vi "3.0.0_Power_Tunings & AW_Performance_Test_ECO_&_BOOST.vi"(7 "Data in":T1, 8 "error in (no error)":errorcluster, 9 "AllControls In":T2, 10 "?":T4, 11 "Message Queue out":T5) -> (0 "error out":errorcluster, 1 "Flow":string, 2 "Data":T4, 3 "Message Queue Out":T5, 5 "Data out":T1)   [LabVIEW 2017]
uses:
  Depends/AMC/subVIs/TypeDefs/amc_Message Queue.ctl
  Depends/AMC/subVIs/TypeDefs/amc_Message.ctl
  Depends/Tools/Keyed Array/Tools_KeyedArray KeyedArray.ctl
  Ctrls/Data.ctl
  DIPC 692 Daemon API/typdef/airwatt tune parameter.ctl
  Ctrls/AllControls.ctl
  Ctrls/CSV_Data.ctl
  DIPC 692 Daemon API/typdef/calibration.ctl
panel:
  out "Array":T3[](array[typedef])
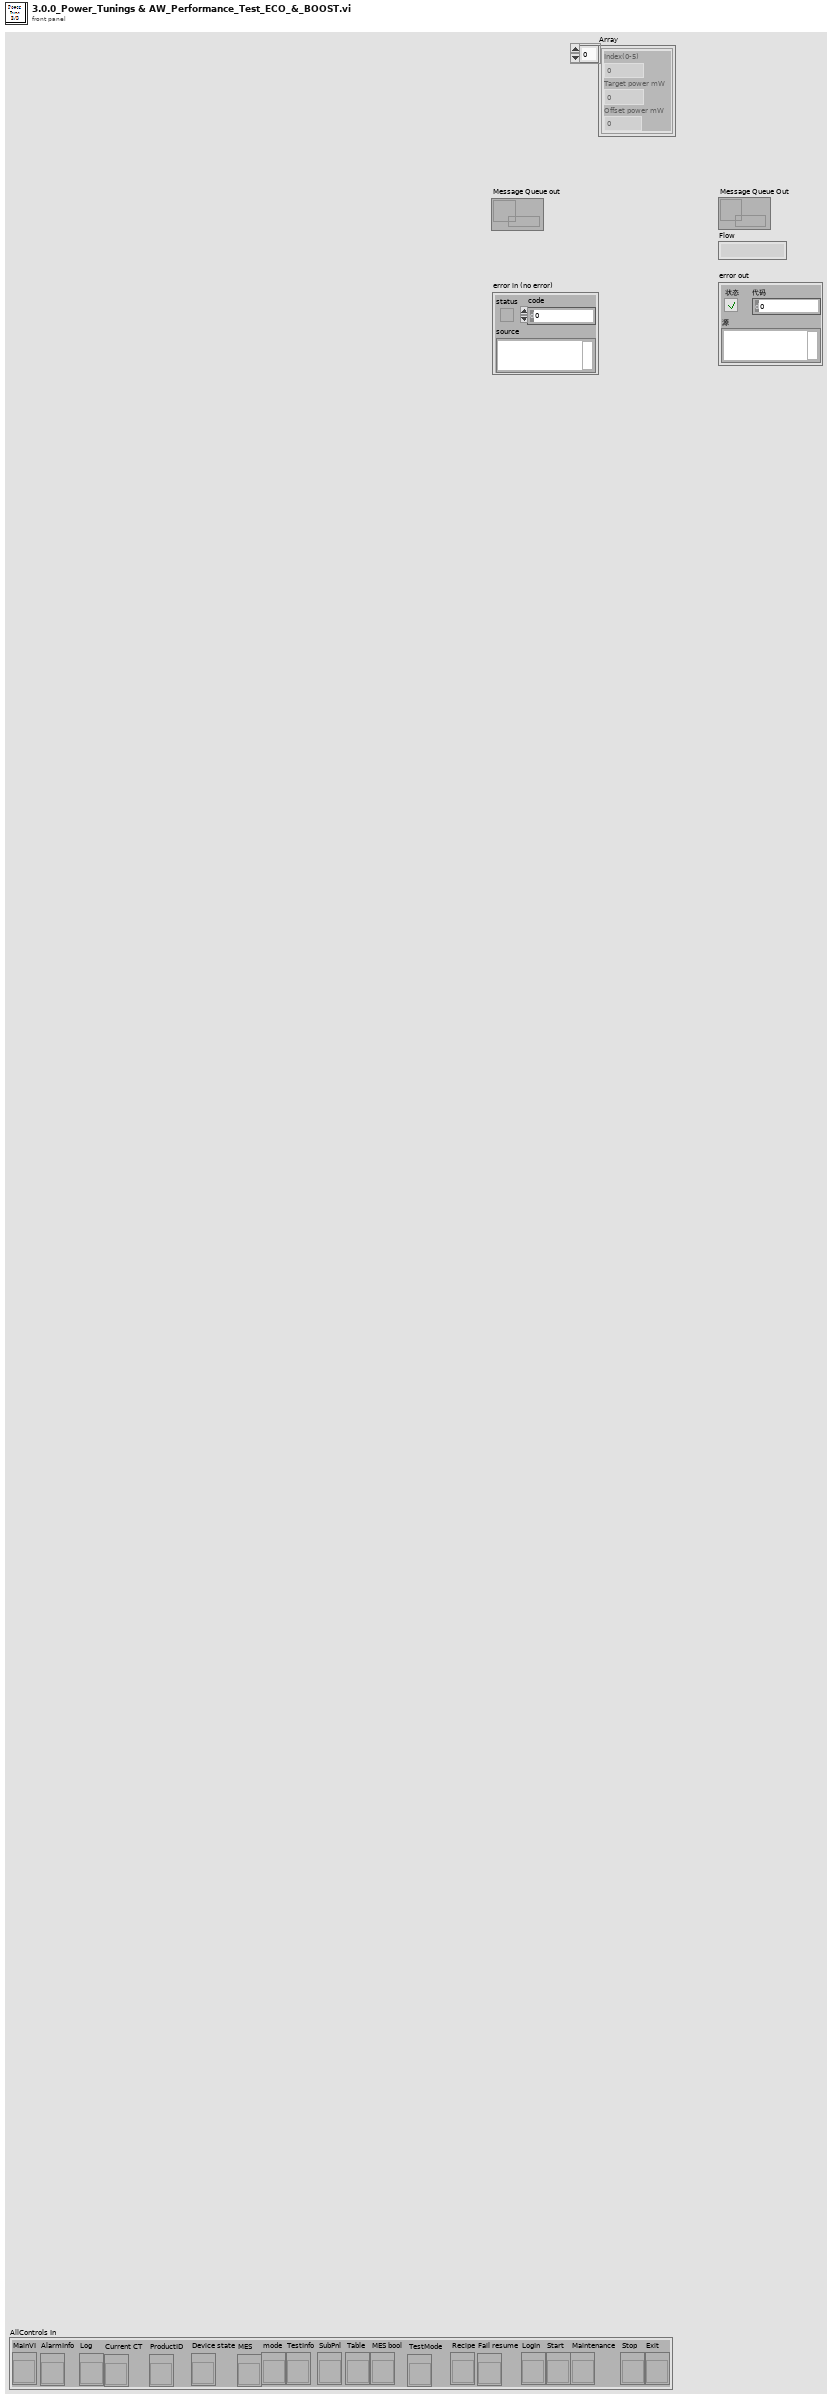
[diagram p1: front panel]
types:
  T1 = typedef "CSV_Data.ctl" = cluster{"Initialisation":cluster{"LMT - Connect UUT (con COM)":string, "LMT - Software Version (rrel)":string, "LMT - Write SKU file (wskuc)":string, "LMT - SKU file name":string, "Connect UUT DDM":string, "Read DDM EOL Timestamp - Mode":string, "Read DDM EOL Timestamp - Timestamp":string, "Read DDM EOL Timestamp - Rig ID":string, "Read DDM EOL Timestamp - Passmark ID":string, "Read DDM EOL Timestamp - Passmark Rev":string, "Software Version before flashing":string, "Read Hardware Serial":string, "UUT DDM SN":string, "Compare DDM SN with MES SN":string, "Backup PCBA Calibration EEPROM Response - CAL":string, "Flash Firmware Version":string, "Check SW Version":string, "Read DDM SW Version after flashing":string, "Set SKU Config":string, "Ready Status":string, "Set Device Mode to EOL":string, "DDM Parameter - Voltage":string, "DDM Parameter - Current":string, "DDM Parameter - Power":string, "DDM Parameter - Speed":string, "DDM Parameter - Pressure":string, "Tester Parameter - Voltage":string, "Tester Parameter - Current":string, "Tester Parameter - Power":string, "Tester Parameter - Ambient Pressure":string, "Tester Parameter - Ambient Temperature":string, "Calculated Parameter - DDM Pressure Corrected":string, "Calculated Parameter - DDM Real Power":string, "Calculated Parameter - Delta V":string}, "BEMF_Calibration":cluster{"Calibration Result - eol_cold_bemf_temp":string, "DDM Ambient Temp":string, "Restriction Plate Diameter":string, "Calibration Result - eol_bemf_mp_cold_coef_a":string, "Calibration Result - eol_bemf_mp_cold_coef_b":string, "Calibration Result - eol_bemf_mp_cold_coef_c":string, "Calibration Result - eol_bemf_lsi_cold_ref_coeffs":string, "Get - Calibration Result - eol_bemf_lsi_speed":string, "Get - Calibration Result - eol_bemf_lsi_integral_0":string, "Calibration Result - eol_bemf_lsi_integral_1":string, "Get - Calibration Result - eol_bemf_lsi_integral_2":string, "Get - Calibration Result - eol_cold_bemf":string, "Get - Calibration Result - eol_cold_bemf_fisf":string, "Finalise Calibration":string, "Compare -Calibration Result - eol_cold_bemf":string, "Compare -Calibration Result - eol_cold_bemf_fisf":string}, "ECO":cluster{"Reset Power Tune":string, "Reset BEMF FISF Calibration":string, "Restriction Plate Diameter":string, "ECO - Stabilisation Time":string, "ECO - DDM Parameter - Voltage":string, "ECO - DDM Parameter - Current":string, "ECO - DDM Parameter - Power":string, "ECO - DDM Parameter - Measured Power":string, "ECO - DDM Parameter - Speed":string, "ECO - DDM Parameter - Pressure":string, "ECO - Tester Parameter - Voltage":string, "ECO - Tester Parameter - Current":string, "ECO - Tester Parameter - Power":string, "ECO - Tester Parameter - Ambient Pressure":string, "ECO - Tester Parameter - Ambient Temperature":string, "ECO - Tester Parameter - Ambient Humidity":string, "ECO - Calculated Parameter - DDM Pressure Corrected":string, "ECO - Calculated Parameter - DDM Real Power":string, "ECO - Calculated Parameter - Delta V":string, "ECO - Calculated Parameter - Flowrate":string, "ECO - Calculated Parameter - Airwatt":string, "ECO - Formula":string, "PT ECO - Power Tune Mode Status":string}, "BOOST":cluster{"Restriction Plate Diameter":string, "BOOST - Stabilisation Time":string, "BOOST - DDM Parameter - Voltage":string, "BOOST - DDM Parameter - Current":string, "BOOST - DDM Parameter - Power":string, "BOOST - DDM Parameter - Measured Power":string, "BOOST - DDM Parameter - Speed":string, "BOOST - DDM Parameter - Pressure":string, "BOOST - Tester Parameter - Voltage":string, "BOOST - Tester Parameter - Current":string, "BOOST - Tester Parameter - Power":string, "BOOST - Tester Parameter - Ambient Pressure":string, "BOOST - Tester Parameter - Ambient Temperature":string, "BOOST - Tester Parameter - Ambient Humidity":string, "BOOST - Calculated Parameter - DDM Pressure Corrected":string, "BOOST - Calculated Parameter - DDM Real Power":string, "BOOST - Calculated Parameter - Delta V":string, "BOOST - Calculated Parameter - Flowrate":string, "BOOST - Calculated Parameter - Airwatt":string, "BOOST - Get AM Presence":string, "Air Muscle Turn Off Status":string, "BOOST - Air Muscle Calculated Parameter - Airwatt B":string, "BOOST - Air Muscle Calculate Airwatt Delta":string, "PT BOOST - Power Tune Mode Status":string, "Finalise Calibration":string, "ECO - Get AW Calibration value":string, "BOOST - Get AW Calibration value":string}, "MAX":cluster{"Restriction Plate Diameter":string, "MAX - Stabilisation Time":string, "Get Average Delta Tmag (LSIdelta_FISFdelta_LSItmag_FISFtmag_IIRtmag)":string, "Get Average Delta Tmag FISF":string, "MAX - DDM Parameter - Voltage":string, "MAX - DDM Parameter - Current":string, "MAX - DDM Parameter - Power":string, "MAX - DDM Parameter - Measured Power":string, "MAX - DDM Parameter - Speed":string, "MAX - DDM Parameter - Pressure":string, "MAX - Tester Parameter - Voltage":string, "MAX - Tester Parameter - Current":string, "MAX - Tester Parameter - Power":string, "MAX - Tester Parameter - Ambient Pressure":string, "MAX - Tester Parameter - Ambient Temperature":string, "MAX - Tester Parameter - Ambient Humidity":string, "MAX - Calculated Parameter - DDM Pressure Corrected":string, "MAX - Calculated Parameter - DDM Real Power":string, "MAX - Calculated Parameter - Delta V":string, "MAX - Calculated Parameter - Flowrate":string, "MAX - Calculated Parameter - Airwatt":string, "MAX_FISF_Check_Average_Delta_Tmag":string, "MAX - FISF - BEMF Finetune Result":string, "MAX tune - Delta P1":string, "MAX tune - Calculated Parameter - Airwatt":string, "Calculate Delta Airwatts - MAX finetune - Delta P2":string, "MAX finetune - DDM Parameter - Voltage":string, "MAX finetune - DDM Parameter - Current":string, "MAX finetune - DDM Parameter - Power":string, "MAX finetune - DDM Parameter - Measured Power":string, "MAX finetune - DDM Parameter - Speed":string, "MAX finetune - DDM Parameter - Pressure":string, "MAX finetune - Tester Parameter - Voltage":string, "MAX finetune - Tester Parameter - Current":string, "MAX finetune - Tester Parameter - Power":string, "MAX finetune - Tester Parameter - Ambient Pressure":string, "MAX finetune - Tester Parameter - Ambient Temperature":string, "MAX finetune - Tester Parameter - Ambient Humidity":string, "MAX finetune - Calculated Parameter - DDM Pressure Corrected":string, "MAX finetune - Calculated Parameter - DDM Real Power":string, "MAX finetune - Calculated Parameter - Delta V":string, "MAX finetune - Calculated Parameter - Flowrate":string, "MAX finetune - Calculated Parameter - Airwatt":string, "Check Derate Result":string, "Delta Tmag FISF":string, "Get Hot BEMF Result":string, "Calculate delta Pressure":string, "Finalise Calibration":string, "Calculate & Check Delta BEMF":string, "Delta P Airwatts Value":string}, "LL":cluster{"DDM Ambient Temp":string, "Restriction Plate Diameter":string, "LL - DDM Parameter - Voltage":string, "LL - DDM Parameter - Current":string, "LL - DDM Parameter - Power":string, "LL - DDM Parameter - Measured Power":string, "LL - DDM Parameter - Speed":string, "LL - DDM Parameter - Pressure":string, "LL - Tester Parameter - Voltage":string, "LL - Tester Parameter - Current":string, "LL - Tester Parameter - Power":string, "LL - DDM Real Power":string, "LL - Calibrate Task Detect LL":string}, "HL":cluster{"HL - DDM Parameter - Voltage":string, "HL - DDM Parameter - Current":string, "HL - DDM Parameter - Power":string, "HL - DDM Parameter - Measured Power":string, "HL - DDM Parameter - Speed":string, "HL - DDM Parameter - Pressure":string, "HL - Tester Parameter - Voltage":string, "HL - Tester Parameter - Current":string, "HL - Tester Parameter - Power":string, "HL - DDM Real Power":string, "HL - Calibrate Task Detect HL":string}, "LH":cluster{"Restriction Plate Diameter":string, "LH - DDM Parameter - Voltage":string, "LH - DDM Parameter - Current":string, "LH - DDM Parameter - Power":string, "LH - DDM Parameter - Measured Power":string, "LH - DDM Parameter - Speed":string, "LH - DDM Parameter - Pressure":string, "LH - Tester Parameter - Voltage":string, "LH - Tester Parameter - Current":string, "LH - Tester Parameter - Power":string, "LH - DDM Real Power":string, "LH - Calibrate Task Detect LH":string}, "HH":cluster{"HH - DDM Parameter - Voltage":string, "HH - DDM Parameter - Current":string, "HH - DDM Parameter - Power":string, "HH - DDM Parameter - Measured Power":string, "HH - DDM Parameter - Speed":string, "HH - DDM Parameter - Pressure":string, "HH - Tester Parameter - Voltage":string, "HH - Tester Parameter - Current":string, "HH - Tester Parameter - Power":string, "HH - DDM Real Power":string, "HH - Calibrate Task Detect HH":string}, "Inlet Blockage Calibration":cluster{"Inlet Blockage Calibration - DDM Parameter - Voltage":string, "Inlet Blockage Calibration - DDM Parameter - Current":string, "Inlet Blockage Calibration - DDM Parameter - Power":string, "Inlet Blockage Calibration - DDM Parameter - Measured Power":string, "Inlet Blockage Calibration - DDM Parameter - Speed":string, "Inlet Blockage Calibration - DDM Parameter - Pressure":string, "Inlet Blockage Calibration - Tester Parameter - Voltage":string, "Inlet Blockage Calibration - Tester Parameter - Current":string, "Inlet Blockage Calibration - Tester Parameter - Power":string, "Inlet Blockage Calibration - DDM Real Power":string, "Calibration Inlet Blockage_E":string, "Finalise Calibration":string, "Get Task Detect LL":string, "Get Task Detect HL":string, "Get Task Detect LH":string, "Get Task Detect HH":string, "Calibration Inlet Blockage":string, "Calibration eol cold bemf temp":string}, "GOOD":cluster{"GOOD UNIT - Clear EEPROM Error Log":string, "GOOD UNIT - Write Product Timestamp - Mode":string, "GOOD UNIT - Write Product Timestamp - Timestamp":string, "GOOD UNIT - Write Product Timestamp - Rig ID":string, "GOOD UNIT - Write Product Timestamp - Passmark ID":string, "GOOD UNIT - Write Product Timestamp - Passmark Rev":string, "GOOD UNIT - Set Device Mode to PROD":string, "GOOD UNIT - Backup PCBA Calibration EEPROM Response":string, "GOOD UNIT - Check Security Bit":string, "GOOD UNIT - Set Calibration Lock":string, "GOOD UNIT - Get_Calibration_Lock":string, "GOOD UNIT - Disconnect UUT":string}, "NG":cluster{"NG UNIT - Read NVM Error":string, "NG UNIT - Set Device Mode to FCT":string, "NG UNIT - Backup PCBA Calibration EEPROM Response - CAL":string, "NG UNIT - Backup PCBA Calibration EEPROM Response - ERROR":string, "NG UNIT - Backup PCBA Calibration EEPROM Response - USAGE":string, "NG UNIT - Disconnect UUT":string}, "SN":string, "Table":string[][], "Count":cluster{"Total":i32, "OK":i32, "NG":i32, "Yield":dbl}, "Start Time":timestamp, "daemon reference":refnum<k5>, "CT":dbl, "Config":string[][], "OK/NG":bool, "Station ID":string, "MES DDM SN":string, "MES PCBA SN":string, "Retest":string, "Variant":string, "Initialisation_Status":cluster{"LMT - Connect UUT (con COM)":string, "LMT - Software Version (rrel)":string, "LMT - Write SKU file (wskuc)":string, "LMT - SKU file name":string, "Connect UUT DDM":string, "Read DDM EOL Timestamp - Mode":string, "Read DDM EOL Timestamp - Timestamp":string, "Read DDM EOL Timestamp - Rig ID":string, "Read DDM EOL Timestamp - Passmark ID":string, "Read DDM EOL Timestamp - Passmark Rev":string, "Software Version before flashing":string, "Read Hardware Serial":string, "UUT DDM SN":string, "Compare DDM SN with MES SN":string, "Backup PCBA Calibration EEPROM Response - CAL":string, "Flash Firmware Version":string, "Check SW Version":string, "Read DDM SW Version after flashing":string, "Set SKU Config":string, "Ready Status":string, "Set Device Mode to EOL":string, "DDM Parameter - Voltage":string, "DDM Parameter - Current":string, "DDM Parameter - Power":string, "DDM Parameter - Speed":string, "DDM Parameter - Pressure":string, "Tester Parameter - Voltage":string, "Tester Parameter - Current":string, "Tester Parameter - Power":string, "Tester Parameter - Ambient Pressure":string, "Tester Parameter - Ambient Temperature":string, "Calculated Parameter - DDM Pressure Corrected":string, "Calculated Parameter - DDM Real Power":string, "Calculated Parameter - Delta V":string}, "BEMF_Calibration_Status":cluster{"Calibration Result - eol_cold_bemf_temp":string, "DDM Ambient Temp":string, "Restriction Plate Diameter":string, "Calibration Result - eol_bemf_mp_cold_coef_a":string, "Calibration Result - eol_bemf_mp_cold_coef_b":string, "Calibration Result - eol_bemf_mp_cold_coef_c":string, "Calibration Result - eol_bemf_lsi_cold_ref_coeffs":string, "Get - Calibration Result - eol_bemf_lsi_speed":string, "Get - Calibration Result - eol_bemf_lsi_integral_0":string, "Calibration Result - eol_bemf_lsi_integral_1":string, "Get - Calibration Result - eol_bemf_lsi_integral_2":string, "Get - Calibration Result - eol_cold_bemf":string, "Get - Calibration Result - eol_cold_bemf_fisf":string, "Finalise Calibration":string, "Compare -Calibration Result - eol_cold_bemf":string, "Compare -Calibration Result - eol_cold_bemf_fisf":string}, "ECO_Status":cluster{"Reset Power Tune":string, "Reset BEMF FISF Calibration":string, "Restriction Plate Diameter":string, "ECO - Stabilisation Time":string, "ECO - DDM Parameter - Voltage":string, "ECO - DDM Parameter - Current":string, "ECO - DDM Parameter - Power":string, "ECO - DDM Parameter - Measured Power":string, "ECO - DDM Parameter - Speed":string, "ECO - DDM Parameter - Pressure":string, "ECO - Tester Parameter - Voltage":string, "ECO - Tester Parameter - Current":string, "ECO - Tester Parameter - Power":string, "ECO - Tester Parameter - Ambient Pressure":string, "ECO - Tester Parameter - Ambient Temperature":string, "ECO - Tester Parameter - Ambient Humidity":string, "ECO - Calculated Parameter - DDM Pressure Corrected":string, "ECO - Calculated Parameter - DDM Real Power":string, "ECO - Calculated Parameter - Delta V":string, "ECO - Calculated Parameter - Flowrate":string, "ECO - Calculated Parameter - Airwatt":string, "ECO - Formula":string, "PT ECO - Power Tune Mode Status":string}, "BOOST_Status":cluster{"Restriction Plate Diameter":string, "BOOST - Stabilisation Time":string, "BOOST - DDM Parameter - Voltage":string, "BOOST - DDM Parameter - Current":string, "BOOST - DDM Parameter - Power":string, "BOOST - DDM Parameter - Measured Power":string, "BOOST - DDM Parameter - Speed":string, "BOOST - DDM Parameter - Pressure":string, "BOOST - Tester Parameter - Voltage":string, "BOOST - Tester Parameter - Current":string, "BOOST - Tester Parameter - Power":string, "BOOST - Tester Parameter - Ambient Pressure":string, "BOOST - Tester Parameter - Ambient Temperature":string, "BOOST - Tester Parameter - Ambient Humidity":string, "BOOST - Calculated Parameter - DDM Pressure Corrected":string, "BOOST - Calculated Parameter - DDM Real Power":string, "BOOST - Calculated Parameter - Delta V":string, "BOOST - Calculated Parameter - Flowrate":string, "BOOST - Calculated Parameter - Airwatt":string, "BOOST - Get AM Presence":string, "Air Muscle Turn Off Status":string, "BOOST - Air Muscle Calculated Parameter - Airwatt B":string, "BOOST - Air Muscle Calculate Airwatt Delta":string, "PT BOOST - Power Tune Mode Status":string, "Finalise Calibration":string, "ECO - Get AW Calibration value":string, "BOOST - Get AW Calibration value":string}, "MAX_Status":cluster{"Restriction Plate Diameter":string, "MAX - Stabilisation Time":string, "Get Average Delta Tmag (LSIdelta_FISFdelta_LSItmag_FISFtmag_IIRtmag)":string, "Get Average Delta Tmag FISF":string, "MAX - DDM Parameter - Voltage":string, "MAX - DDM Parameter - Current":string, "MAX - DDM Parameter - Power":string, "MAX - DDM Parameter - Measured Power":string, "MAX - DDM Parameter - Speed":string, "MAX - DDM Parameter - Pressure":string, "MAX - Tester Parameter - Voltage":string, "MAX - Tester Parameter - Current":string, "MAX - Tester Parameter - Power":string, "MAX - Tester Parameter - Ambient Pressure":string, "MAX - Tester Parameter - Ambient Temperature":string, "MAX - Tester Parameter - Ambient Humidity":string, "MAX - Calculated Parameter - DDM Pressure Corrected":string, "MAX - Calculated Parameter - DDM Real Power":string, "MAX - Calculated Parameter - Delta V":string, "MAX - Calculated Parameter - Flowrate":string, "MAX - Calculated Parameter - Airwatt":string, "MAX_FISF_Check_Average_Delta_Tmag":string, "MAX - FISF - BEMF Finetune Result":string, "MAX tune - Delta P1":string, "MAX tune - Calculated Parameter - Airwatt":string, "Calculate Delta Airwatts - MAX finetune - Delta P2":string, "MAX finetune - DDM Parameter - Voltage":string, "MAX finetune - DDM Parameter - Current":string, "MAX finetune - DDM Parameter - Power":string, "MAX finetune - DDM Parameter - Measured Power":string, "MAX finetune - DDM Parameter - Speed":string, "MAX finetune - DDM Parameter - Pressure":string, "MAX finetune - Tester Parameter - Voltage":string, "MAX finetune - Tester Parameter - Current":string, "MAX finetune - Tester Parameter - Power":string, "MAX finetune - Tester Parameter - Ambient Pressure":string, "MAX finetune - Tester Parameter - Ambient Temperature":string, "MAX finetune - Tester Parameter - Ambient Humidity":string, "MAX finetune - Calculated Parameter - DDM Pressure Corrected":string, "MAX finetune - Calculated Parameter - DDM Real Power":string, "MAX finetune - Calculated Parameter - Delta V":string, "MAX finetune - Calculated Parameter - Flowrate":string, "MAX finetune - Calculated Parameter - Airwatt":string, "Check Derate Result":string, "Delta Tmag FISF":string, "Get Hot BEMF Result":string, "Calculate delta Pressure":string, "Finalise Calibration":string, "Calculate & Check Delta BEMF":string, "Delta P Airwatts Value":string}, "LL_Status":cluster{"DDM Ambient Temp":string, "Restriction Plate Diameter":string, "LL - DDM Parameter - Voltage":string, "LL - DDM Parameter - Current":string, "LL - DDM Parameter - Power":string, "LL - DDM Parameter - Measured Power":string, "LL - DDM Parameter - Speed":string, "LL - DDM Parameter - Pressure":string, "LL - Tester Parameter - Voltage":string, "LL - Tester Parameter - Current":string, "LL - Tester Parameter - Power":string, "LL - DDM Real Power":string, "LL - Calibrate Task Detect LL":string}, "HL_Status":cluster{"HL - DDM Parameter - Voltage":string, "HL - DDM Parameter - Current":string, "HL - DDM Parameter - Power":string, "HL - DDM Parameter - Measured Power":string, "HL - DDM Parameter - Speed":string, "HL - DDM Parameter - Pressure":string, "HL - Tester Parameter - Voltage":string, "HL - Tester Parameter - Current":string, "HL - Tester Parameter - Power":string, "HL - DDM Real Power":string, "HL - Calibrate Task Detect HL":string}, "LH_Status":cluster{"Restriction Plate Diameter":string, "LH - DDM Parameter - Voltage":string, "LH - DDM Parameter - Current":string, "LH - DDM Parameter - Power":string, "LH - DDM Parameter - Measured Power":string, "LH - DDM Parameter - Speed":string, "LH - DDM Parameter - Pressure":string, "LH - Tester Parameter - Voltage":string, "LH - Tester Parameter - Current":string, "LH - Tester Parameter - Power":string, "LH - DDM Real Power":string, "LH - Calibrate Task Detect LH":string}, "HH_Status":cluster{"HH - DDM Parameter - Voltage":string, "HH - DDM Parameter - Current":string, "HH - DDM Parameter - Power":string, "HH - DDM Parameter - Measured Power":string, "HH - DDM Parameter - Speed":string, "HH - DDM Parameter - Pressure":string, "HH - Tester Parameter - Voltage":string, "HH - Tester Parameter - Current":string, "HH - Tester Parameter - Power":string, "HH - DDM Real Power":string, "HH - Calibrate Task Detect HH":string}, "Inlet Blockage Calibration_Status":cluster{"Inlet Blockage Calibration - DDM Parameter - Voltage":string, "Inlet Blockage Calibration - DDM Parameter - Current":string, "Inlet Blockage Calibration - DDM Parameter - Power":string, "Inlet Blockage Calibration - DDM Parameter - Measured Power":string, "Inlet Blockage Calibration - DDM Parameter - Speed":string, "Inlet Blockage Calibration - DDM Parameter - Pressure":string, "Inlet Blockage Calibration - Tester Parameter - Voltage":string, "Inlet Blockage Calibration - Tester Parameter - Current":string, "Inlet Blockage Calibration - Tester Parameter - Power":string, "Inlet Blockage Calibration - DDM Real Power":string, "Calibration Inlet Blockage_E":string, "Finalise Calibration":string, "Get Task Detect LL":string, "Get Task Detect HL":string, "Get Task Detect LH":string, "Get Task Detect HH":string, "Calibration Inlet Blockage":string, "Calibration eol cold bemf temp":string}, "GOOD_Status":cluster{"GOOD UNIT - Clear EEPROM Error Log":string, "GOOD UNIT - Write Product Timestamp - Mode":string, "GOOD UNIT - Write Product Timestamp - Timestamp":string, "GOOD UNIT - Write Product Timestamp - Rig ID":string, "GOOD UNIT - Write Product Timestamp - Passmark ID":string, "GOOD UNIT - Write Product Timestamp - Passmark Rev":string, "GOOD UNIT - Set Device Mode to PROD":string, "GOOD UNIT - Backup PCBA Calibration EEPROM Response":string, "GOOD UNIT - Check Security Bit":string, "GOOD UNIT - Set Calibration Lock":string, "GOOD UNIT - Get_Calibration_Lock":string, "GOOD UNIT - Disconnect UUT":string}, "NG_Status":cluster{"NG UNIT - Read NVM Error":string, "NG UNIT - Set Device Mode to FCT":string, "NG UNIT - Backup PCBA Calibration EEPROM Response - CAL":string, "NG UNIT - Backup PCBA Calibration EEPROM Response - ERROR":string, "NG UNIT - Backup PCBA Calibration EEPROM Response - USAGE":string, "NG UNIT - Disconnect UUT":string}, "SKU":string, "Plate_Diameter":string, "Alarm":string}
  T2 = typedef "AllControls.ctl" = cluster{"MainVI":refnum<vi>, "AlarmInfo":refnum<vi>, "Log":refnum<vi>, "Current CT":refnum<vi>, "ProductID":refnum<vi>, "Device state":refnum<vi>, "MES":refnum<vi>, "mode":refnum<vi>, "TestInfo":refnum<vi>, "SubPnl":refnum<vi>, "Table":refnum<vi>, "MES bool":refnum<vi>, "TestMode":refnum<vi>, "Recipe":refnum<vi>, "Fail resume":refnum<vi>, "LogIn":refnum<vi>, "Start":refnum<vi>, "Maintenance":refnum<vi>, "Stop":refnum<vi>, "Exit":refnum<vi>}
  T3 = typedef "airwatt tune parameter.ctl" = cluster{"Index(0-5)":i64, "Target power mW":i64, "Offset power mW":i64}
  T4 = typedef "Data.ctl" = cluster{"Initialisation":cluster{"DDM_Parameter":dbl[], "DDM_Parameter_status":bool[], "Get_Tester_Parameter":dbl[], "Get_Tester_Parameter_status":bool[], "Cal_Tester_Parameter":dbl[], "Cal_Tester_Parameter_status":bool[], "sw_version_before_status":bool, "sw_version_after_status":bool, "Set_SKU_Config_With_LMT_status":bool, "FCT_timestamp_status":bool, "LMT_Connect_to_UUT_status":bool}, "BEMF_Calibration":cluster{"Read_ambient_temperature":dbl, "Calibration_Vaule":dbl[], "Calibration_Vaule _B":dbl[], "Calibration_Vaule_status":bool[], "Calibration_Vaule_B_status":bool[]}, "ECO":cluster{"DDM_Parameter":dbl[], "DDM_Parameter_status":bool[], "Get_Tester_Parameter":dbl[], "Get_Tester_Parameter_status":bool[], "Cal_Tester_Parameter":dbl[], "Cal_Tester_Parameter_status":bool[], "DDM_Parameter_after_power_tune":dbl[], "Get_Tester_Parameter_after_power_tune":dbl[], "Cal_Tester_Parameter_after_power_tune":dbl[], "Cal_Tester_Parameter_after_power_tune_status":bool[], "Delta_P":dbl}, "BOOST":cluster{"DDM_Parameter":dbl[], "DDM_Parameter_status":bool[], "Get_Tester_Parameter":dbl[], "Get_Tester_Parameter_status":bool[], "Cal_Tester_Parameter":dbl[], "Cal_Tester_Parameter_status":bool[], "DDM_Parameter_after_power_tune":dbl[], "Get_Tester_Parameter_after_power_tune":dbl[], "Cal_Tester_Parameter_after_power_tune":dbl[], "Cal_Tester_Parameter_after_power_tune_status":bool[], "airwatts_am_off":dbl, "AW_Delta_(AM_on_and_off)":dbl, "AW_Delta_(AM_on_and_off)_Status":bool, "Delta_P":dbl}, "MAX":cluster{"Average_Tmag_Data":cluster{"LSI Delta in degC":dbl, "FISF Delta in degc":dbl, "LSI Tmag in degC":dbl, "Fisf Tmag in degC":dbl, "IIR Tmag in degC":dbl}, "DDM_Parameter":dbl[], "DDM_Parameter_status":bool[], "Get_Tester_Parameter":dbl[], "Get_Tester_Parameter_status":bool[], "Cal_Tester_Parameter":dbl[], "BEMF_Finetune":cluster{"eol_bemf_mp_cold_coef_c":dbl, "eol_cold_bemf_fisf_offset":dbl}, "AW_Tune":cluster{"delta_P1":dbl, "delta_P_Setting":dbl}, "DDM_Parameter_after_Airwatts_Tune":dbl[], "Get_Tester_Parameter_after_Airwatts_Tune":dbl[], "Cal_Tester_Parameter_after_Airwatts_Tune":dbl[], "DDM_Parameter_after_Airwatts_Finetune":dbl[], "Get_Tester_Parameter_after_Airwatts_Finetune":dbl[], "Cal_Tester_Parameter_after_Airwatts_Finetune":dbl[], "AW_Finetune":cluster{"delta_P2":dbl, "delta_P_Setting":dbl}, "Delta_Tmag_after_tune":cluster{"LSI Delta in degC":dbl, "FISF Delta in degc":dbl, "LSI Tmag in degC":dbl, "Fisf Tmag in degC":dbl, "IIR Tmag in degC":dbl}, "Hot Bemf in mV":dbl, "DDM_Pressure":dbl, "Delta_Pressure":dbl, " Cold Bemf in mV":dbl, " delta Bemf":dbl, " delta p":dbl, "Delta_Pressure_status":bool, " delta Bemf_status":bool, "LSI Delta in degC_status":bool, "FISF Delta in degc_status":bool, "Max_check_derate_status_status":bool, "Average_All_data":dbl[][], "Average_Tmag_Data_status":bool[], "Average_Tmag_Data_after_tune_status":bool[], "Cal_Tester_Parameter_status":bool[], "Cal_Tester_Parameter_status_after_Airwatts_Tune":bool[], "Cal_Tester_Parameter_status_after_Airwatts_FineTune":bool[]}, "Task_Detect_Calib":cluster{"LL":cluster{"DDM_Parameter":dbl[], "DDM_Parameter_status":bool[], "Get_Tester_Parameter":dbl[], "Get_Tester_Parameter_status":bool[], "Set_task_detect_A":dbl, "Set_task_detect_A_Status":bool}, "HL":cluster{"DDM_Parameter":dbl[], "DDM_Parameter_status":bool[], "Get_Tester_Parameter":dbl[], "Get_Tester_Parameter_status":bool[], "Set_task_detect_B":dbl, "Set_task_detect_B_Status":bool}, "LH":cluster{"DDM_Parameter":dbl[], "DDM_Parameter_status":bool[], "Get_Tester_Parameter":dbl[], "Get_Tester_Parameter_status":bool[], "Set_task_detect_C":dbl, "Set_task_detect_C_Status":bool}, "HH":cluster{"DDM_Parameter":dbl[], "DDM_Parameter_status":bool[], "Get_Tester_Parameter":dbl[], "Get_Tester_Parameter_status":bool[], "Set_task_detect_D":dbl, "Read_and_check_calibration_Status":bool[], "Set_task_detect_D_Status":bool}, "Get_eol_inlet_blockage_E":dbl, "Calib_vaule":cluster{"Get_task_detect_LL":dbl, "Get_task_detect_HL":dbl, "Get_task_detect_LH":dbl, "Get_task_detect_HH":dbl, "eol_inlet_blockage":dbl, "eol_code_bemf_temp":dbl}, "calibrated temp":dbl, "Inlet_Blockage_Calibration":cluster{"DDM_Parameter":dbl[], "DDM_Parameter_status":bool[], "Get_Tester_Parameter":dbl[], "Get_Tester_Parameter_status":bool[]}, "Get_eol_inlet_blockage_E_Status":bool}, "good":cluster{"Write_Product_TS":cluster{"TIMESTAMP":i64, "RIG_ID":i64, "PASSMARK_ID":i64, "PASSMARK_REV":i64}, "Read_Product_TS":cluster{"TIMESTAMP":i64, "RIG_ID":i64, "PASSMARK_ID":i64, "PASSMARK_REV":i64}, "Good_Check_Secuity_Bit_Stauts":bool}}
  T5 = typedef "amc_Message Queue.ctl" = refnum<queue>
  T6 = typedef "HD Config.ctl" = cluster{" PC":cluster{"PC Address":u8[], "PC Port":i32}, "FCO":cluster{"COM":refnum<visa-resource-name>, "Baudrate":u32}, "DC Power ":cluster{"COM":refnum<visa-resource-name>, "Baudrate":u32}, "PW3336":cluster{"COM":refnum<visa-resource-name>, "Baudrate":u32}, "Lefoo":cluster{"COM":refnum<visa-resource-name>, "Baudrate":u32}, "AI Model":cluster{"COM":refnum<visa-resource-name>, "Baudrate":u32}, "DIPC":cluster{"COM":refnum<visa-resource-name>}, "NFC":cluster{"IP Address":string, "Port":u16, "Retry":u16}, "Motor":cluster{"COM":refnum<visa-resource-name>, "Baudrate":u32}, "Fail_resume_mode":bool, "GRR":bool}
  T7 = typedef "calibration.ctl" = string
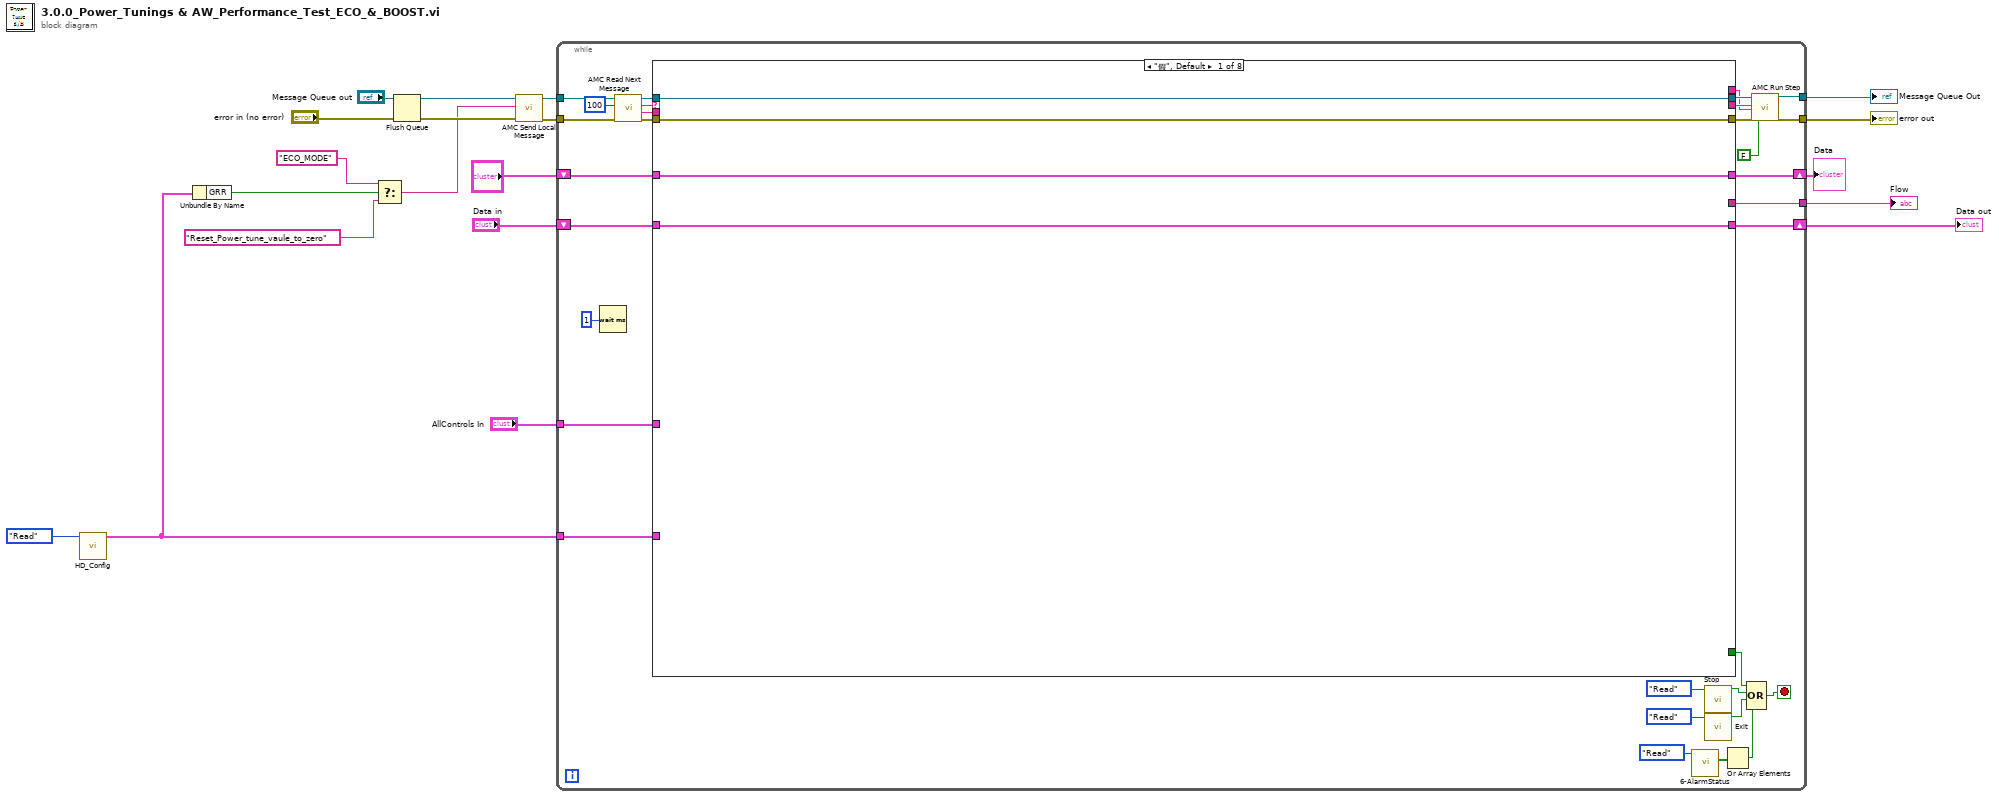
[diagram p0: block diagram]
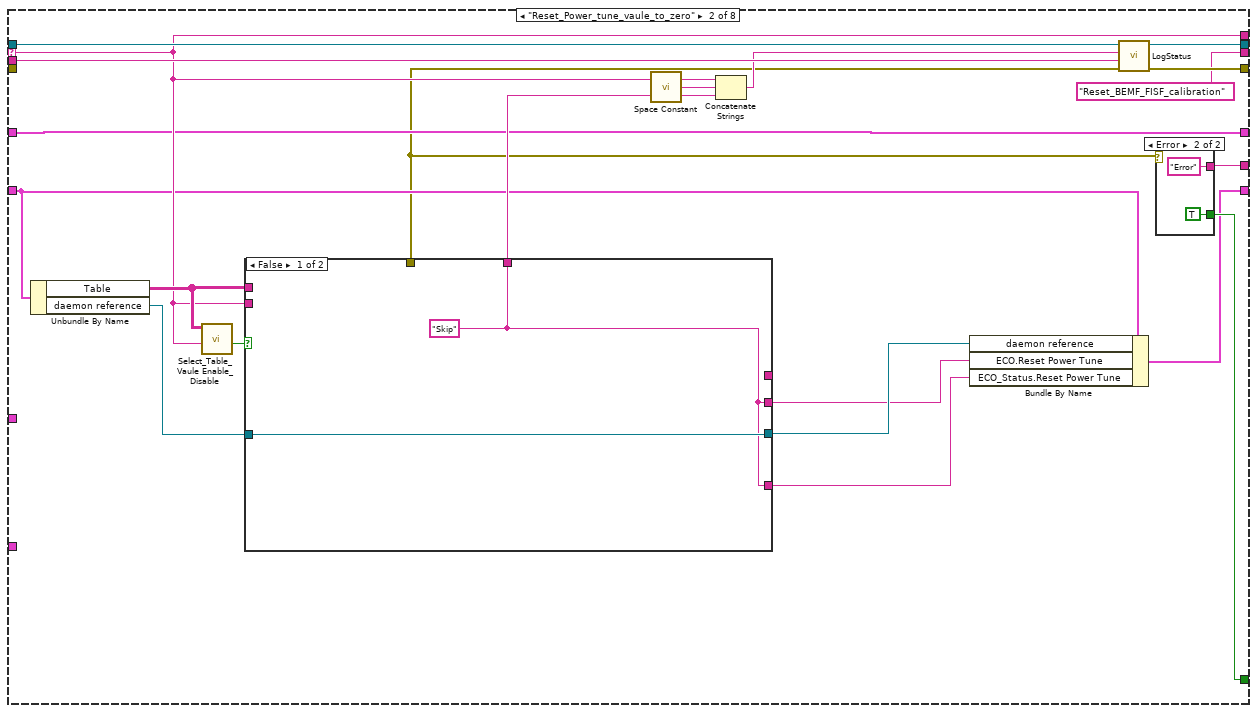
[diagram p2: hidden frame]
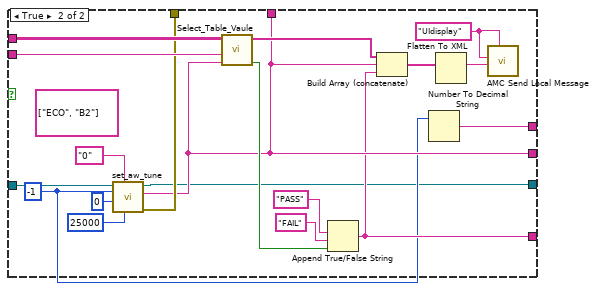
[diagram p4: hidden frame]
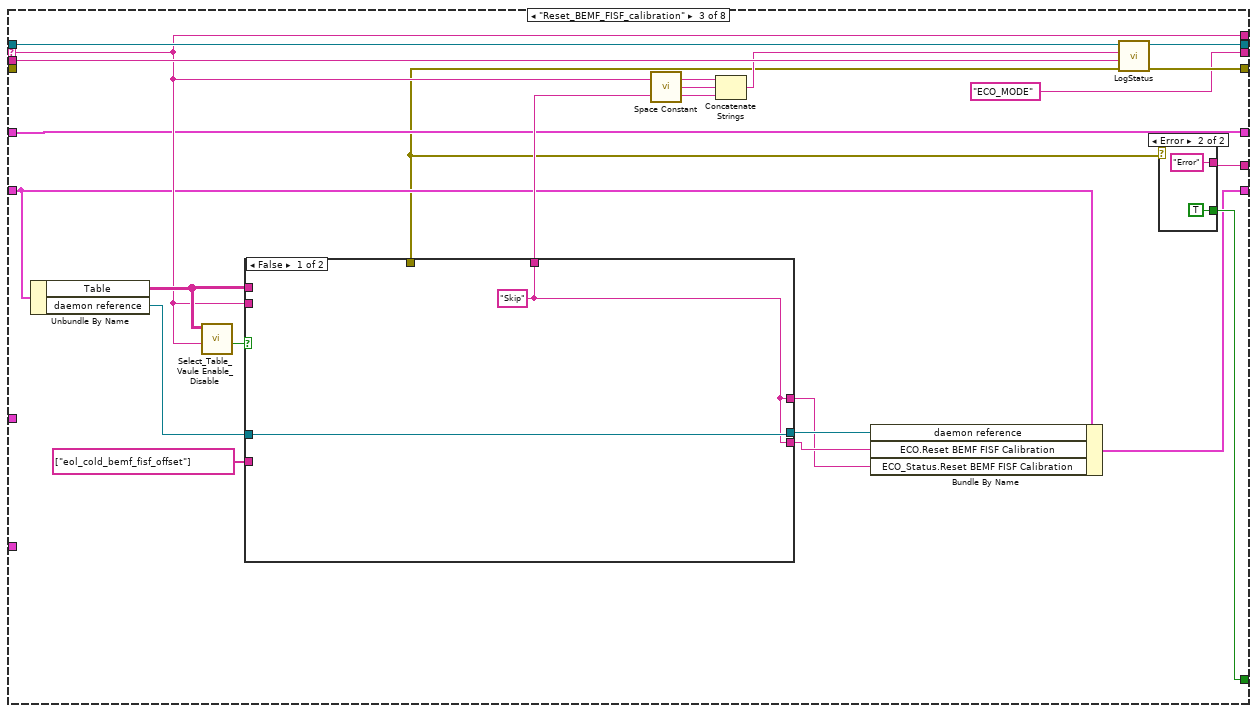
[diagram p5: hidden frame]
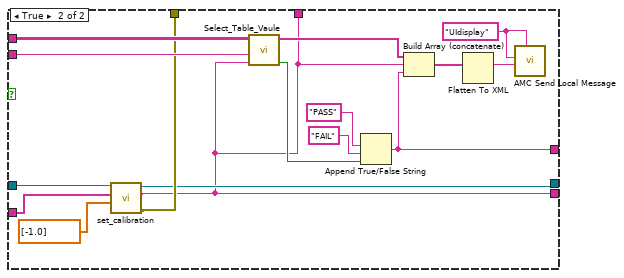
[diagram p7: hidden frame]
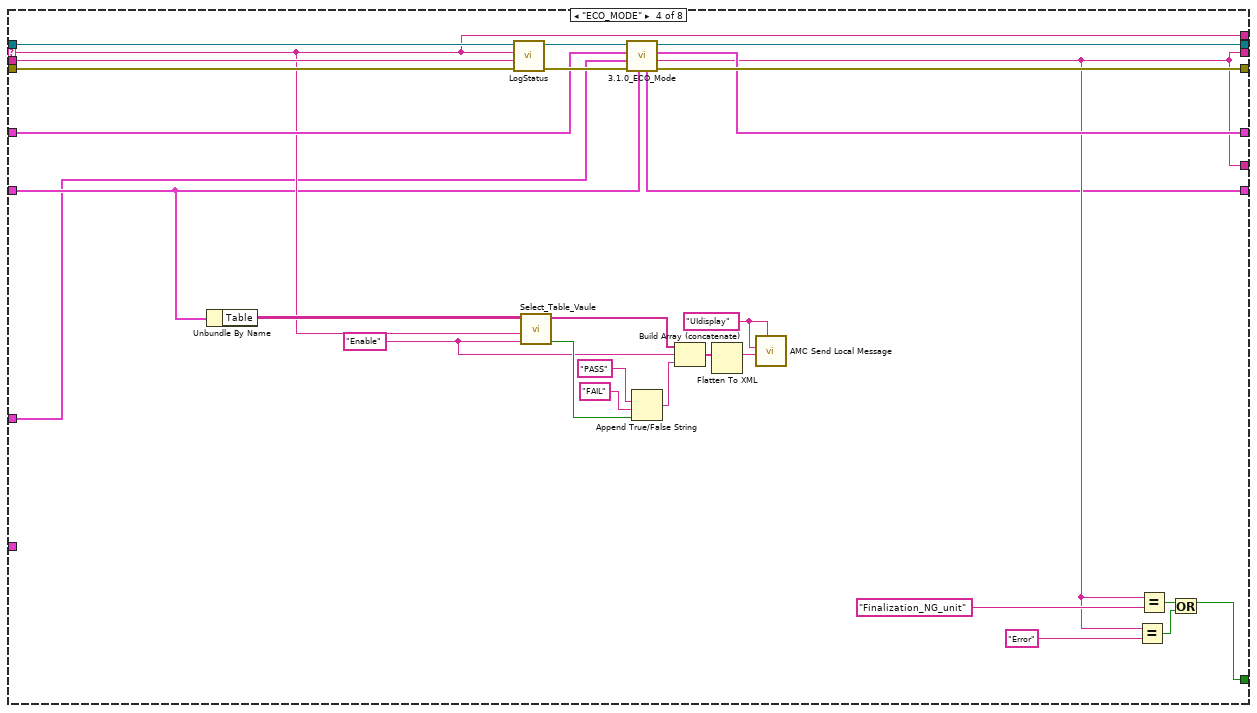
[diagram p8: hidden frame]
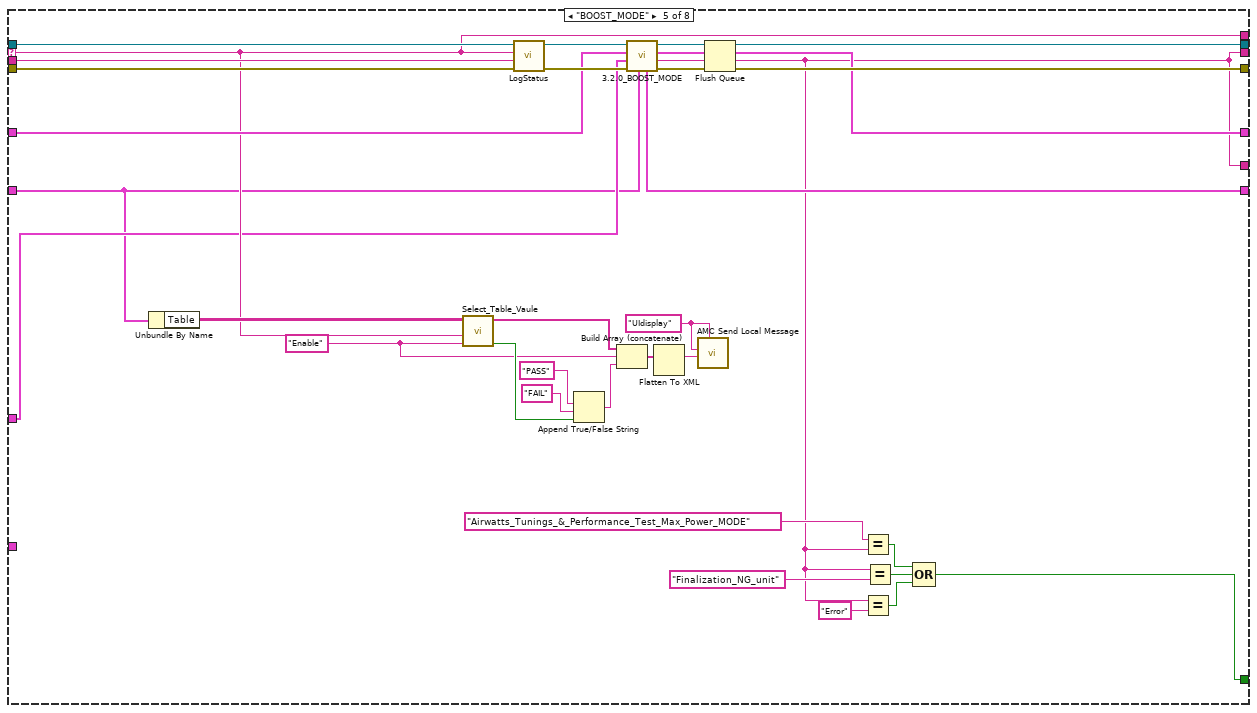
[diagram p9: hidden frame]
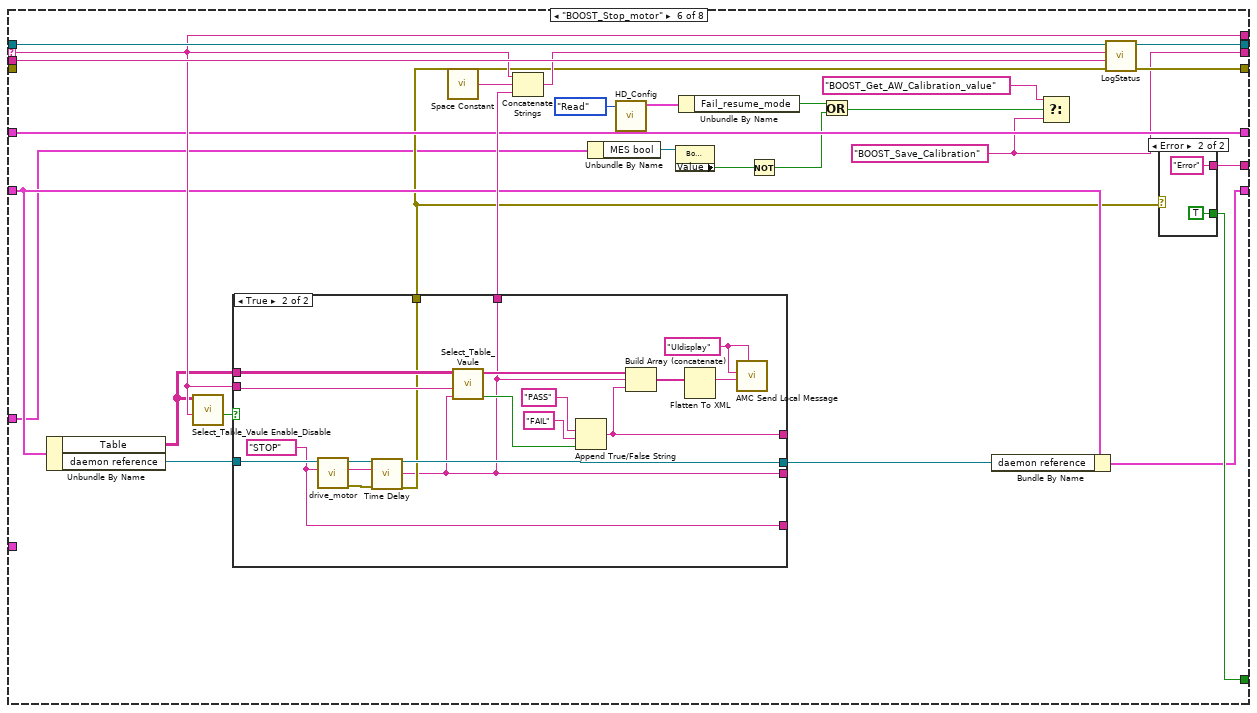
[diagram p10: hidden frame]
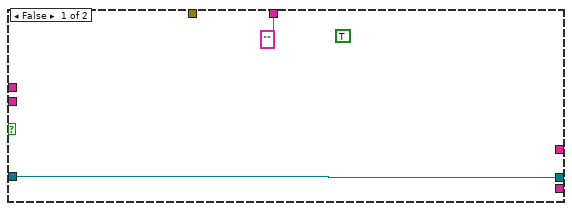
[diagram p12: hidden frame]
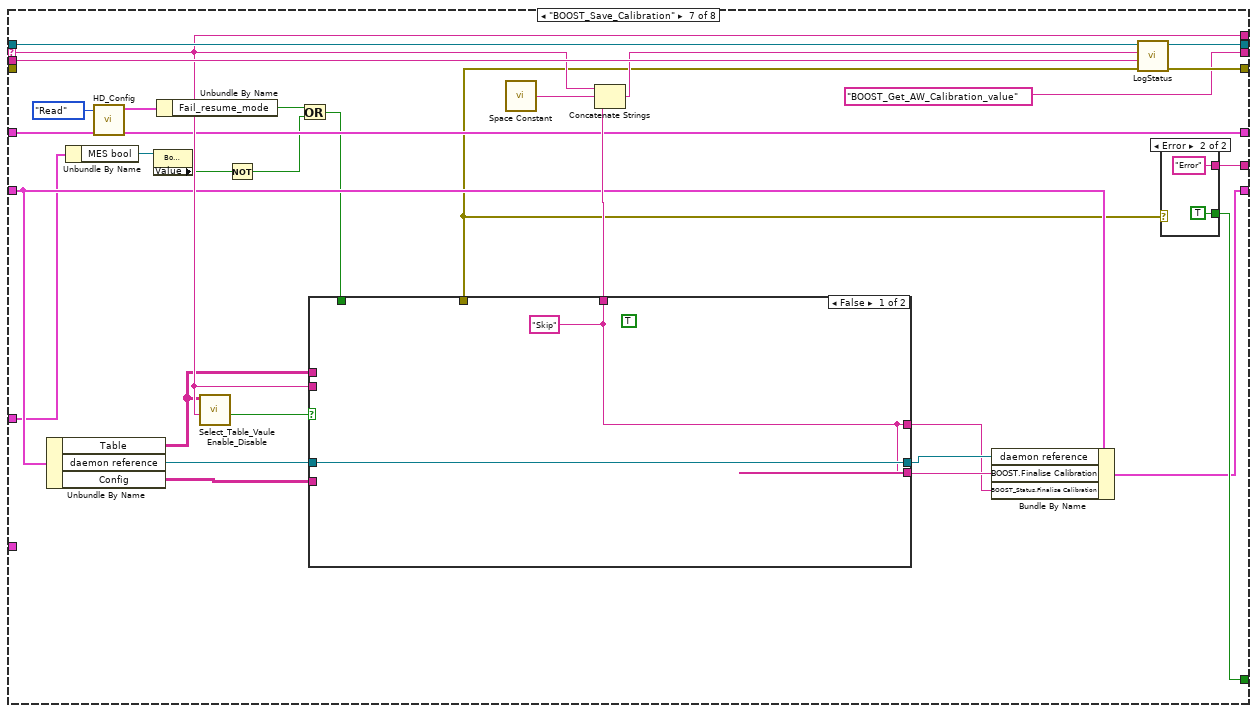
[diagram p13: hidden frame]
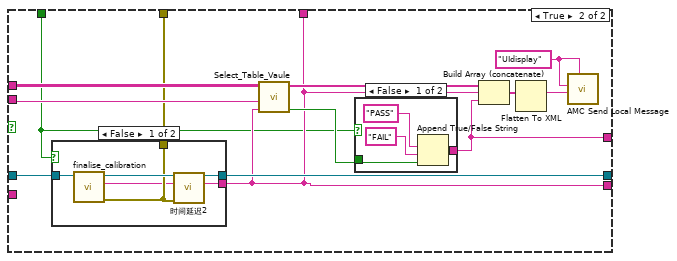
[diagram p15: hidden frame]
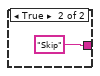
[diagram p16: hidden frame]
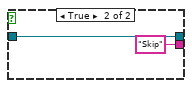
[diagram p17: hidden frame]
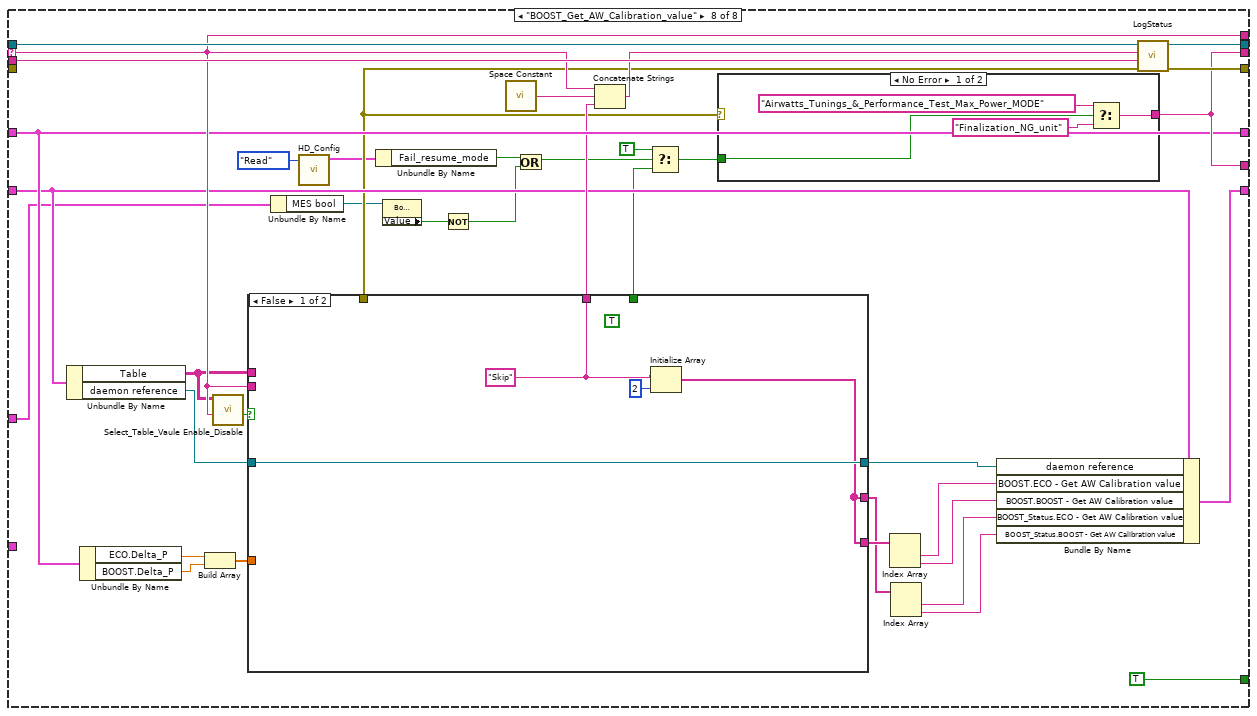
[diagram p18: hidden frame]
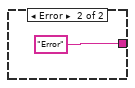
[diagram p19: hidden frame]
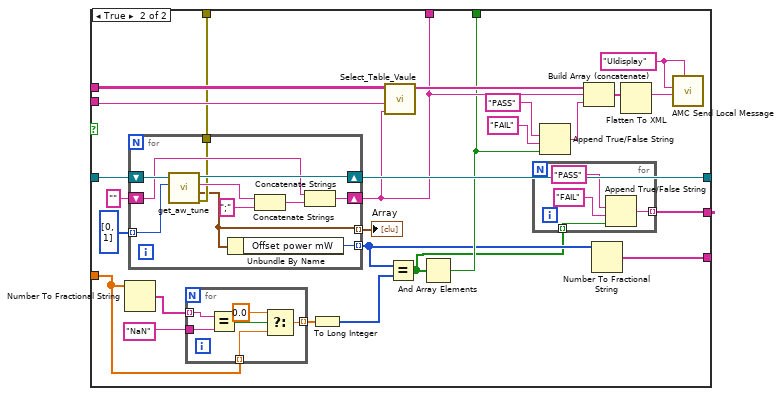
[diagram p20: hidden frame]
diagram:
  n1 = call "HD_Config.vi"("Step"=enum16{"Initial", "Write", "Read"}."Read") -> ("HD Config out"=w5:T6)  [unwired: 9 in, 1 out]
  n2 = Unbundle By Name(w5) -> ("GRR"=w4:bool)
  n3 = Select(t="ECO_MODE", s=w4, f="Reset_Power_tune_vaule_to_zero" ("Message Name")) -> (s? t:f=w2:string)
  n4 = Flush Queue(queue="Message Queue out") -> (queue out=w11:T5)  [unwired: 1 in, 2 out]
  n5 = call "AMC Send Local Message.vi"("error in (no error)"="error in (no error)", "Message Name"=w2, "Message Queue in"=w11) -> ("error out"=w17:errorcluster, "Message Queue out"=w18:T5)  [unwired: 7 in]
  n6 = while {
    tunnel: w18 -> [w50]
    tunnel: [w46] -> w10
    tunnel: w17 -> [w44]
    tunnel: [w41] -> w9
    shift-right: [w37] -> w14
    shift-left: "?" -> [w38]
    tunnel: w5 -> [w36]
    tunnel: [w32] -> w12
    shift-right: [w24] -> w7
    shift-left: "Data in" -> [w23]
    tunnel: "AllControls In" -> [w25]
    stop <- w26 stop-if-true
    n7 = Wait (ms)(milliseconds to wait=u32 1 ("等待时间（毫秒）")) -> ()  [unwired: 1 out]
    n8 = call "AMC Read Next Message.vi"("error in (no error)"=w44, "timeout (1ms)"=100, "Message Queue in"=w50) -> ("error out"=w43:errorcluster, "Message Value"=w34:string, "Message Name"=w48:string, "Message Queue out"=w49:T5)  [unwired: 1 in, 4 out]
    n9 = case shown="\"假\", Default" w48 {
      selector: w48 -> [_ w66 w110 w147 w179 w218 w266 w333]
      tunnel: w49 -> [w54 w74 w118 w162 w193 w224 w273 w338]
      tunnel: [w54 w74 w118 w161 w173 w224 w273 w338] -> w47
      tunnel: w43 -> [w53 _ _ w166 w197 _ _ _]
      tunnel: [w53 w73 w117 w163 w194 w223 w272 w337] -> w42
      tunnel: [_ w63 w106 w143 w174 w214 w261 TRUE] -> w27
      tunnel: w38 -> [w52 w61 w104 w148 w180 w212 w259 w324]
      tunnel: [w52 w61 w104 w160 w191 w212 w259 w324] -> w37
      tunnel: w34 -> [_ w72 w116 w165 w196 w222 w271 w336]
      tunnel: [_ w66 w110 w147 w179 w218 w266 w333] -> w33
      tunnel: w36 -> [_ _ _ _ _ _ _ _]
      tunnel: [_ "Reset_BEMF_FISF_calibration" "ECO_MODE" w145 w168 w198 "BOOST_Get_AW_Calibration_value" w327] -> w35
      tunnel: [_ w64 w107 w145 w168 w215 w262 w327] -> w32
      tunnel: w25 -> [_ _ _ w139 w172 w200 w246 w311]
      tunnel: [w51 w57 w100 w140 w171 w208 w255 w318] -> w24
      tunnel: w23 -> [w51 w60 w103 w141 w170 w211 w258 w322]
      frame "假", Default {
      }
      frame "Reset_Power_tune_vaule_to_zero" {
        n10 = Unbundle By Name(w60) -> ("Table"=w67:string[][], "daemon reference"=w62:refnum<k5>)
        n11 = call "Select_Table_Vaule Enable_Disable.vi"("Action"=w66, "Table"=w67) -> ("Enable"=w65:bool)  [unwired: 8 in, 1 out]
        n12 = case shown="False" w65 {
          tunnel: [w77 w83] -> w68
          tunnel: w67 -> [_ w90]
          tunnel: w66 -> [_ w89]
          tunnel: w62 -> [w78 w88]
          tunnel: [_ w87] -> w59
          tunnel: [w77 w83] -> w56
          tunnel: [w77 w82] -> w55
          tunnel: [_ w80] -> _
          tunnel: [w78 w79] -> w58
          frame False {
            w77 = "Skip" ("response")
          }
          frame True {
            w81 = -1 ("Index")
            (unwired) string[] ["ECO", "B2"]
            w96 = "UIdisplay" ("Process (\"\" - local)")
            n13 = call "set_aw_tune.vi"("timeout (25000ms)"=25000, "Power Mode or Target Power in W"="0", "Offset Power mW"=0, "Index"=w81, "daemon reference in"=w88) -> ("error out"=w87:errorcluster, "response"=w83:string, "daemon reference out"=w79:refnum<k5>)  [unwired: 3 in, 1 out]
            n14 = call "Select_Table_Vaule.vi"("Vaule"=w83, "Action"=w89, "Table"=w90) -> ("Result"=w91:bool, "vaule"=w97:string[])  [unwired: 7 in]
            n15 = Append True/False String(1:w91, 2:"FAIL" ("真字符串"), 3:"PASS" ("真字符串")) -> (0:w82:string)  [unwired: 1 in]
            n16 = Build Array (concatenate)(w97, w83, w82) -> (w95:string[])
            n17 = Number To Decimal String(number=w81) -> (decimal integer string=w80:string)  [unwired: 1 in]
            n18 = Flatten To XML(anything=w95) -> (xml string=w94:string)
            n19 = call "AMC Send Local Message.vi"("Process (\"\" - local)"=w96, "Message Value"=w94, "Message Name"=w96) -> ()  [unwired: 7 in, 2 out]
          }
        }
        n20 = call <vilib>:"Space Constant.vi"() -> ("String"=w69:string)
        n21 = Concatenate Strings(w66, w69, w68) -> (w70:string)
        n22 = Bundle By Name(cluster=w60, "daemon reference"=w58, "ECO.Reset Power Tune"=w56, "ECO_Status.Reset Power Tune"=w55) -> (w57:T1)
        n23 = call "LogStatus.vi"("error in (no error)"=w59, "last message"=w72, "message"=w70) -> ("error  out"=w73:errorcluster)  [unwired: 8 in]
        n24 = case shown="Error" w59 {
          tunnel: [_ TRUE] -> w63
          tunnel: [_ "Error"] -> w64
          frame No Error {
          }
          frame Error {
          }
        }
      }
      frame "Reset_BEMF_FISF_calibration" {
        n25 = Unbundle By Name(w103) -> ("Table"=w111:string[][], "daemon reference"=w108:refnum<k5>)
        n26 = call "Select_Table_Vaule Enable_Disable.vi"("Action"=w110, "Table"=w111) -> ("Enable"=w109:bool)  [unwired: 8 in, 1 out]
        n27 = case shown="False" w109 {
          tunnel: [w121 w124] -> w112
          tunnel: w111 -> [_ w131]
          tunnel: w110 -> [_ w130]
          tunnel: w108 -> [w122 w128]
          tunnel: [_ w127] -> w102
          tunnel: T7[] ["eol_cold_bemf_fisf_offset"] ("calibration") -> [_ w126]
          tunnel: [w122 w125] -> w101
          tunnel: [w121 w124] -> w99
          tunnel: [w121 w123] -> w98
          frame False {
            w121 = "Skip" ("response")
          }
          frame True {
            w137 = "UIdisplay" ("Process (\"\" - local)")
            n28 = call "set_calibration.vi"("values"=dbl[] [-1.0], "calibration"=w126, "daemon reference in"=w128) -> ("error out"=w127:errorcluster, "response"=w124:string, "daemon reference out"=w125:refnum<k5>)  [unwired: 5 in, 1 out]
            n29 = call "Select_Table_Vaule.vi"("Vaule"=w124, "Action"=w130, "Table"=w131) -> ("Result"=w132:bool, "vaule"=w138:string[])  [unwired: 7 in]
            n30 = Append True/False String(1:w132, 2:"FAIL" ("真字符串"), 3:"PASS" ("真字符串")) -> (0:w123:string)  [unwired: 1 in]
            n31 = Build Array (concatenate)(w138, w124, w123) -> (w136:string[])
            n32 = Flatten To XML(anything=w136) -> (xml string=w135:string)
            n33 = call "AMC Send Local Message.vi"("Process (\"\" - local)"=w137, "Message Value"=w135, "Message Name"=w137) -> ()  [unwired: 7 in, 2 out]
          }
        }
        n34 = call <vilib>:"Space Constant.vi"() -> ("String"=w113:string)
        n35 = Concatenate Strings(w110, w113, w112) -> (w114:string)
        n36 = Bundle By Name(cluster=w103, "daemon reference"=w101, "ECO.Reset BEMF FISF Calibration"=w99, "ECO_Status.Reset BEMF FISF Calibration"=w98) -> (w100:T1)
        n37 = call "LogStatus.vi"("error in (no error)"=w102, "last message"=w116, "message"=w114) -> ("error  out"=w117:errorcluster)  [unwired: 8 in]
        n38 = case shown="Error" w102 {
          tunnel: [_ TRUE] -> w106
          tunnel: [_ "Error"] -> w107
          frame No Error {
          }
          frame Error {
          }
        }
      }
      frame "ECO_MODE" {
        w150 = "UIdisplay" ("Process (\"\" - local)")
        w146 = "Enable" ("元素")
        n39 = Unbundle By Name(w141) -> ("Table"=w149:string[][])
        n40 = call "LogStatus.vi"("error in (no error)"=w166, "last message"=w165, "message"=w147) -> ("error  out"=w164:errorcluster)  [unwired: 8 in]
        n41 = call "Select_Table_Vaule.vi"("Vaule"=w146, "Action"=w147, "Table"=w149) -> ("Result"=w157:bool, "vaule"=w156:string[])  [unwired: 7 in]
        n42 = call "3.1.0_ECO_Mode.vi"("Data in"=w141, "error in (no error)"=w164, "AllControls In"=w139, 10:w148, "Message Queue out"=w162) -> ("error out"=w163:errorcluster, "Flow"=w145:string, "Data"=w160:T4, "Message Queue Out"=w161:T5, "Data out"=w140:T1)  [unwired: 2 in]
        n43 = Append True/False String(1:w157, 2:"FAIL" ("真字符串"), 3:"PASS" ("真字符串")) -> (0:w155:string)  [unwired: 1 in]
        n44 = Build Array (concatenate)(w156, w146, w155) -> (w153:string[])
        n45 = Flatten To XML(anything=w153) -> (xml string=w154:string)
        n46 = call "AMC Send Local Message.vi"("Process (\"\" - local)"=w150, "Message Value"=w154, "Message Name"=w150) -> ()  [unwired: 7 in, 2 out]
        n47 = Equal?(x=w145, y="Error") -> (x = y?=w142:bool)
        n48 = Equal?(x=w145, y="Finalization_NG_unit") -> (x = y?=w158:bool)
        n49 = Or(x=w158, y=w142) -> (x .or. y?=w143:bool)
      }
      frame "BOOST_MODE" {
        w183 = "UIdisplay" ("Process (\"\" - local)")
        w181 = "Enable" ("元素")
        n50 = Unbundle By Name(w170) -> ("Table"=w182:string[][])
        n51 = call "Select_Table_Vaule.vi"("Vaule"=w181, "Action"=w179, "Table"=w182) -> ("Result"=w190:bool, "vaule"=w189:string[])  [unwired: 7 in]
        n52 = call "LogStatus.vi"("error in (no error)"=w197, "last message"=w196, "message"=w179) -> ("error  out"=w195:errorcluster)  [unwired: 8 in]
        n53 = Append True/False String(1:w190, 2:"FAIL" ("真字符串"), 3:"PASS" ("真字符串")) -> (0:w188:string)  [unwired: 1 in]
        n54 = Build Array (concatenate)(w189, w181, w188) -> (w186:string[])
        n55 = call "3.2.0_BOOST_MODE.vi"("Data in"=w170, "error in (no error)"=w195, "AllControls In"=w172, 10:w180, "Message Queue out"=w193) -> ("error out"=w194:errorcluster, "Flow"=w168:string, "Data"=w191:T4, "Message Queue Out"=w192:T5, "Data out"=w171:T1)  [unwired: 2 in]
        n56 = Flatten To XML(anything=w186) -> (xml string=w187:string)
        n57 = call "AMC Send Local Message.vi"("Process (\"\" - local)"=w183, "Message Value"=w187, "Message Name"=w183) -> ()  [unwired: 7 in, 2 out]
        n58 = Flush Queue(queue=w192) -> (queue out=w173:T5)  [unwired: 1 in, 2 out]
        n59 = Equal?(x="Airwatts_Tunings_&_Performance_Test_Max_Power_MODE", y=w168) -> (x = y?=w167:bool)
        n60 = Equal?(x=w168, y="Error") -> (x = y?=w175:bool)
        n61 = Equal?(x=w168, y="Finalization_NG_unit") -> (x = y?=w177:bool)
        n62 = Compound Arithmetic op=OR ("复合运算")(w167, w177, w175) -> (w174:bool)
      }
      frame "BOOST_Stop_motor" {
        w198 = "BOOST_Save_Calibration"
        n63 = Unbundle By Name(w211) -> ("Table"=w217:string[][], "daemon reference"=w221:refnum<k5>)
        n64 = call "Select_Table_Vaule Enable_Disable.vi"("Action"=w218, "Table"=w217) -> ("Enable"=w216:bool)  [unwired: 8 in, 1 out]
        n65 = case shown="True" w216 {
          tunnel: w221 -> [w228 w239]
          tunnel: [w228 w238] -> w209
          tunnel: ["" ("software string") w231] -> w213
          tunnel: w218 -> [_ w237]
          tunnel: w217 -> [_ w236]
          tunnel: [_ w233] -> w210
          tunnel: [_ w231] -> _
          tunnel: [_ w230] -> _
          tunnel: [_ w229] -> _
          frame False {
            (unwired) TRUE
          }
          frame True {
            w229 = "STOP" ("Power Mode")
            w244 = "UIdisplay" ("Process (\"\" - local)")
            n66 = call "drive_motor.vi"("Power Mode"=w229, "daemon reference in"=w239) -> ("error out"=w232:errorcluster, "response"=w231:string, "daemon reference out"=w238:refnum<k5>)  [unwired: 6 in, 1 out]
            n67 = call "Time Delay"("error in (no error)"=w232) -> ("error out"=w233:errorcluster)  [unwired: 10 in]
            n68 = call "Select_Table_Vaule.vi"("Vaule"=w231, "Action"=w237, "Table"=w236) -> ("Result"=w234:bool, "vaule"=w235:string[])  [unwired: 7 in]
            n69 = Append True/False String(1:w234, 2:"FAIL" ("真字符串"), 3:"PASS" ("真字符串")) -> (0:w230:string)  [unwired: 1 in]
            n70 = Build Array (concatenate)(w235, w231, w230) -> (w243:string[])
            n71 = Flatten To XML(anything=w243) -> (xml string=w242:string)
            n72 = call "AMC Send Local Message.vi"("Process (\"\" - local)"=w244, "Message Value"=w242, "Message Name"=w244) -> ()  [unwired: 7 in, 2 out]
          }
        }
        n73 = call <vilib>:"Space Constant.vi"() -> ("String"=w220:string)
        n74 = Concatenate Strings(w218, w220, w213) -> (w219:string)
        n75 = Unbundle By Name(w200) -> ("MES bool"=w206:refnum<vi>)
        n76 = call "HD_Config.vi"("Step"=enum16{"Initial", "Write", "Read"}."Read") -> ("HD Config out"=w207:T6)  [unwired: 9 in, 1 out]
        n77 = property class="Bool (严格)"(reference=w206) -> ("Value"=w204:bool)  [unwired: 1 in, 2 out]
        n78 = Unbundle By Name(w207) -> ("Fail_resume_mode"=w205:bool)
        n79 = Not(x=w204) -> (.not. x?=w202:bool)
        n80 = Or(x=w205, y=w202) -> (x .or. y?=w203:bool)
        n81 = Bundle By Name(cluster=w211, "daemon reference"=w209) -> (w208:T1)
        n82 = Select(t="BOOST_Get_AW_Calibration_value", s=w203, f=w198) -> ()  [unwired: 1 out]
        n83 = call "LogStatus.vi"("error in (no error)"=w210, "last message"=w222, "message"=w219) -> ("error  out"=w223:errorcluster)  [unwired: 8 in]
        n84 = case shown="Error" w210 {
          tunnel: [_ TRUE] -> w214
          tunnel: [_ "Error"] -> w215
          frame No Error {
          }
          frame Error {
          }
        }
      }
      frame "BOOST_Save_Calibration" {
        n85 = Unbundle By Name(w258) -> ("Table"=w265:string[][], "daemon reference"=w270:refnum<k5>, "Config"=w263:string[][])
        n86 = Unbundle By Name(w246) -> ("MES bool"=w251:refnum<vi>)
        n87 = call "HD_Config.vi"("Step"=enum16{"Initial", "Write", "Read"}."Read") -> ("HD Config out"=w252:T6)  [unwired: 9 in, 1 out]
        n88 = property class="Bool (严格)"(reference=w251) -> ("Value"=w249:bool)  [unwired: 1 in, 2 out]
        n89 = Unbundle By Name(w252) -> ("Fail_resume_mode"=w250:bool)
        n90 = call "Select_Table_Vaule Enable_Disable.vi"("Action"=w266, "Table"=w265) -> ("Enable"=w264:bool)  [unwired: 8 in, 1 out]
        n91 = Not(x=w249) -> (.not. x?=w248:bool)
        n92 = Or(x=w250, y=w248) -> (x .or. y?=w245:bool)
        n93 = case shown="False" w264 {
          tunnel: w270 -> [w277 w287]
          tunnel: [w277 w286] -> w256
          tunnel: [w276 w280] -> w260
          tunnel: w266 -> [_ w285]
          tunnel: w265 -> [_ w284]
          tunnel: w263 -> [_ _]
          tunnel: [_ w281] -> w257
          tunnel: [w276 w280] -> w254
          tunnel: [w276 w279] -> w253
          tunnel: w245 -> [_ w278]
          frame False {
            w276 = "Skip" ("software string")
            (unwired) TRUE
          }
          frame True {
            w290 = "UIdisplay" ("Process (\"\" - local)")
            n94 = case shown="False" w278 {
              tunnel: w287 -> [w299 w301]
              tunnel: [w298 w301] -> w286
              tunnel: [w297 _] -> w281
              tunnel: [w296 "Skip" ("response")] -> w280
              frame False {
                n95 = call "finalise_calibration.vi"("daemon reference in"=w299) -> ("error out"=w297:errorcluster, "response"=w296:string, "daemon reference out"=w298:refnum<k5>)  [unwired: 7 in, 1 out]
                n96 = call "时间延迟2"("error in (no error)"=w297) -> ()  [unwired: 10 in, 1 out]
              }
              frame True {
              }
            }
            n97 = call "Select_Table_Vaule.vi"("Vaule"=w280, "Action"=w285, "Table"=w284) -> ("Result"=w282:bool, "vaule"=w283:string[])  [unwired: 7 in]
            n98 = case shown="False" w278 {
              tunnel: w282 -> [w292 _]
              tunnel: [w291 "Skip" ("response")] -> w279
              frame False {
                n99 = Append True/False String(1:w292, 2:"FAIL" ("真字符串"), 3:"PASS" ("真字符串")) -> (0:w291:string)  [unwired: 1 in]
              }
              frame True {
              }
            }
            n100 = Build Array (concatenate)(w283, w280, w279) -> (w289:string[])
            n101 = Flatten To XML(anything=w289) -> (xml string=w288:string)
            n102 = call "AMC Send Local Message.vi"("Process (\"\" - local)"=w290, "Message Value"=w288, "Message Name"=w290) -> ()  [unwired: 7 in, 2 out]
          }
        }
        n103 = call <vilib>:"Space Constant.vi"() -> ("String"=w269:string)
        n104 = Concatenate Strings(w266, w269, w260) -> (w268:string)
        n105 = Bundle By Name(cluster=w258, "daemon reference"=w256, "BOOST.Finalise Calibration"=w254, "BOOST_Status.Finalise Calibration"=w253) -> (w255:T1)
        n106 = call "LogStatus.vi"("error in (no error)"=w257, "last message"=w271, "message"=w268) -> ("error  out"=w272:errorcluster)  [unwired: 8 in]
        n107 = case shown="Error" w257 {
          tunnel: [_ TRUE] -> w261
          tunnel: [_ "Error"] -> w262
          frame No Error {
          }
          frame Error {
          }
        }
      }
      frame "BOOST_Get_AW_Calibration_value" {
        n108 = Unbundle By Name(w322) -> ("Table"=w326:string[][], "daemon reference"=w325:refnum<k5>)
        n109 = Unbundle By Name(w324) -> ("ECO.Delta_P"=w331:dbl, "BOOST.Delta_P"=w330:dbl)
        n110 = Build Array(w331, w330) -> (w329:dbl[])
        n111 = call "Select_Table_Vaule Enable_Disable.vi"("Action"=w333, "Table"=w326) -> ("Enable"=w332:bool)  [unwired: 8 in, 1 out]
        n112 = case shown="False" w332 {
          tunnel: w325 -> [w347 w371]
          tunnel: [w347 w370] -> w319
          tunnel: [w346 w361] -> w323
          tunnel: w333 -> [_ w373]
          tunnel: w326 -> [_ w372]
          tunnel: [_ w359] -> w309
          tunnel: w329 -> [_ w353]
          tunnel: [_ w358] -> w321
          tunnel: [w345 w351] -> w320
          tunnel: [w345 w348] -> w304
          frame False {
            w346 = "Skip" ("software string")
            (unwired) TRUE
            n113 = Initialize Array(w346, 2 ("维数大小")) -> (w345:string[])
          }
          frame True {
            w369 = "UIdisplay" ("Process (\"\" - local)")
            n114 = Number To Fractional String(number=w353) -> (F-format string=w355:string[])  [unwired: 3 in]
            n115 = for {
              shift-right: [w394] -> w370
              shift-left: w371 -> [w393]
              tunnel: u32[] [0, 1] -> [w392] mode=indexing
              tunnel: [w391] -> w352 mode=indexing
              shift-right: [w390] -> w361
              shift-left: "" -> [w389]
              tunnel: [w385] -> w358
              tunnel: [w384] -> w356 mode=indexing
              n116 = call "get_aw_tune.vi"("Index"=w392, "daemon reference in"=w393) -> ("error out"=w385:errorcluster, "AW Tune Parameter"=w384:T3, "response"=w388:string, "daemon reference out"=w394:refnum<k5>)  [unwired: 5 in, 1 out]
              n117 = Unbundle By Name(w384) -> ("Offset power mW"=w391:i64)
              n118 = Concatenate Strings(w388, ";" ("字符串")) -> (w386:string)
              n119 = Concatenate Strings(w389, w386) -> (w390:string)
            }
            "Array" <- w356
            n120 = for {
              tunnel: w355 -> [w380] mode=indexing
              tunnel: "NaN" -> [w383]
              tunnel: [w381] -> w357 mode=indexing
              tunnel: w353 -> [w378] mode=indexing
              n121 = Equal?(x=w380, y=w383) -> (x = y?=w382:bool)
              n122 = Select(t=0.0, s=w382, f=w378) -> (s? t:f=w381:dbl)
            }
            n123 = To Long Integer(number=w357) -> (32bit integer=w350:i32[])
            n124 = call "Select_Table_Vaule.vi"("Vaule"=w361, "Action"=w373, "Table"=w372) -> ("vaule"=w363:string[])  [unwired: 7 in, 1 out]
            n125 = Equal?(x=w352, y=w350) -> (x = y?=w349:bool[])
            n126 = And Array Elements(Boolean array=w349) -> (logical AND=w359:bool)
            n127 = for {
              tunnel: w349 -> [w375] mode=indexing
              tunnel: [w374] -> w348 mode=indexing
              n128 = Append True/False String(1:w375, 2:"FAIL" ("真字符串"), 3:"PASS" ("真字符串")) -> (0:w374:string)  [unwired: 1 in]
            }
            n129 = Append True/False String(1:w359, 2:"FAIL" ("真字符串"), 3:"PASS" ("真字符串")) -> (0:w364:string)  [unwired: 1 in]
            n130 = Build Array (concatenate)(w363, w361, w364) -> (w368:string[])
            n131 = Number To Fractional String(number=w352) -> (F-format string=w351:string[])  [unwired: 3 in]
            n132 = Flatten To XML(anything=w368) -> (xml string=w367:string)
            n133 = call "AMC Send Local Message.vi"("Process (\"\" - local)"=w369, "Message Value"=w367, "Message Name"=w369) -> ()  [unwired: 7 in, 2 out]
          }
        }
        n134 = Unbundle By Name(w311) -> ("MES bool"=w316:refnum<vi>)
        n135 = call "HD_Config.vi"("Step"=enum16{"Initial", "Write", "Read"}."Read") -> ("HD Config out"=w317:T6)  [unwired: 9 in, 1 out]
        n136 = Unbundle By Name(w317) -> ("Fail_resume_mode"=w315:bool)
        n137 = property class="Bool (严格)"(reference=w316) -> ("Value"=w314:bool)  [unwired: 1 in, 2 out]
        n138 = Not(x=w314) -> (.not. x?=w313:bool)
        n139 = call <vilib>:"Space Constant.vi"() -> ("String"=w335:string)
        n140 = Or(x=w315, y=w313) -> (x .or. y?=w310:bool)
        n141 = Concatenate Strings(w333, w335, w323) -> (w334:string)
        n142 = Select(t=TRUE, s=w310, f=w309) -> (s? t:f=w308:bool)
        n143 = case shown="No Error" w321 {
          tunnel: w308 -> [w340 _]
          tunnel: [w339 "Error"] -> w327
          frame No Error {
            n144 = Select(t="Airwatts_Tunings_&_Performance_Test_Max_Power_MODE", s=w340, f="Finalization_NG_unit") -> (s? t:f=w339:string)
          }
          frame Error {
          }
        }
        n145 = Index Array(array=w320) -> (element #1=w306:string, element #2=w305:string)  [unwired: 2 in]
        n146 = Index Array(array=w304) -> (element #1=w303:string, element #2=w302:string)  [unwired: 2 in]
        n147 = Bundle By Name(cluster=w322, "daemon reference"=w319, "BOOST.ECO - Get AW Calibration value"=w306, "BOOST.BOOST - Get AW Calibration value"=w305, "BOOST_Status.ECO - Get AW Calibration value"=w303, "BOOST_Status.BOOST - Get AW Calibration value"=w302) -> (w318:T1)
        n148 = call "LogStatus.vi"("error in (no error)"=w321, "last message"=w336, "message"=w334) -> ("error  out"=w337:errorcluster)  [unwired: 8 in]
      }
    }
    n149 = call "6-AlarmStatus.vi"("Step"=enum16{"Initial", "Write", "Read"}."Read") -> ("AlarmValue Out"=w21:bool[])  [unwired: 9 in, 1 out]
    n150 = call "Stop.vi"("Step"=enum16{"Initial", "Write", "Read"}."Read") -> ("Stop Out"=w29:bool)  [unwired: 9 in, 1 out]
    n151 = call "Exit.vi"("Step"=enum16{"Initial", "Write", "Read"}."Read" ("step")) -> ("Exit Out"=w28:bool)  [unwired: 9 in, 1 out]
    n152 = Or Array Elements(Boolean array=w21) -> (logical OR=w20:bool)
    n153 = Compound Arithmetic op=OR(w27, w29, w28, w20) -> (w26:bool)
    n154 = call "AMC Run Step.vi"("Message Queue In"=w47, "Message Name"=w35, "Message Value"=w33, "error in (no error)"=w42, "Mli/Sig"=FALSE) -> ("Message Queue Out"=w46:T5, "error out"=w41:errorcluster)  [unwired: 13 in]
  }
  "Message Queue Out" <- w10
  "error out" <- w9
  "Data" <- w14
  "Flow" <- w12
  "Data out" <- w7
